vi "Get All VIs from Project.vi"(8 "error in (no error)":errorcluster, 11 "Project Path":path) -> (0 "error out":errorcluster, 2 "VI Virtual Paths":string[](array[string]), 3 "Project VIs":path[](array[path]), 5 "Project Name":string)   [LabVIEW 2015, in "SET Project Editor.lvlib"]
doc: "Get All VIs from Project.vi\n\nGet Paths (relative to project root) and Virtual Paths of project VIs\n\nExcluded VIs:\n- Password Protected VIs\n- vi.lib VIs\n- user.lib VIs\n- VIs of type other than Standard or Global"
uses:
  SET Project Editor.lvlib
panel:
  # "Get All VIs from Project.vi\n\nGet Paths (relative to project root) and Virtual Paths of project VIs\n\nExcluded VIs:\n- Password Protected VIs\n- vi.lib VIs\n- user.lib VIs\n- VIs of type other than Standard or Global"
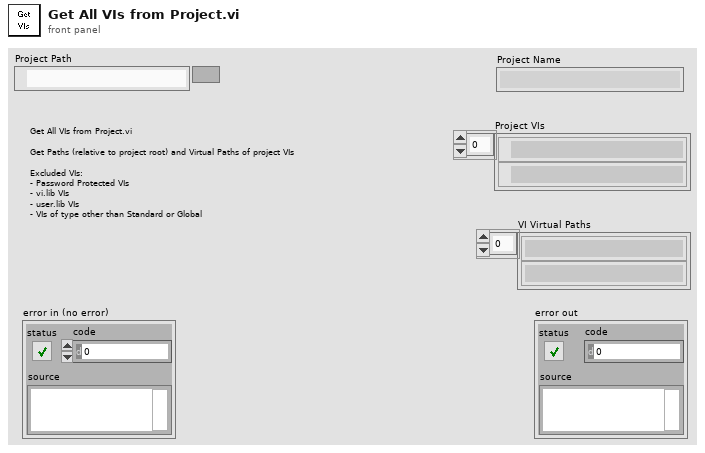
[diagram p1: front panel]
types:
  T1 = enum32{"invalid lock state", "Not Locked", "Locked (No Password)", "Password-protected"}
  T2 = enum32{"invalid VI type", "Standard VI", "Control VI", "Global VI", "Polymorphic VI", "Configuration VI", "SubSystem", "Facade VI", "Method VI", "Statechart Diagram VI"}
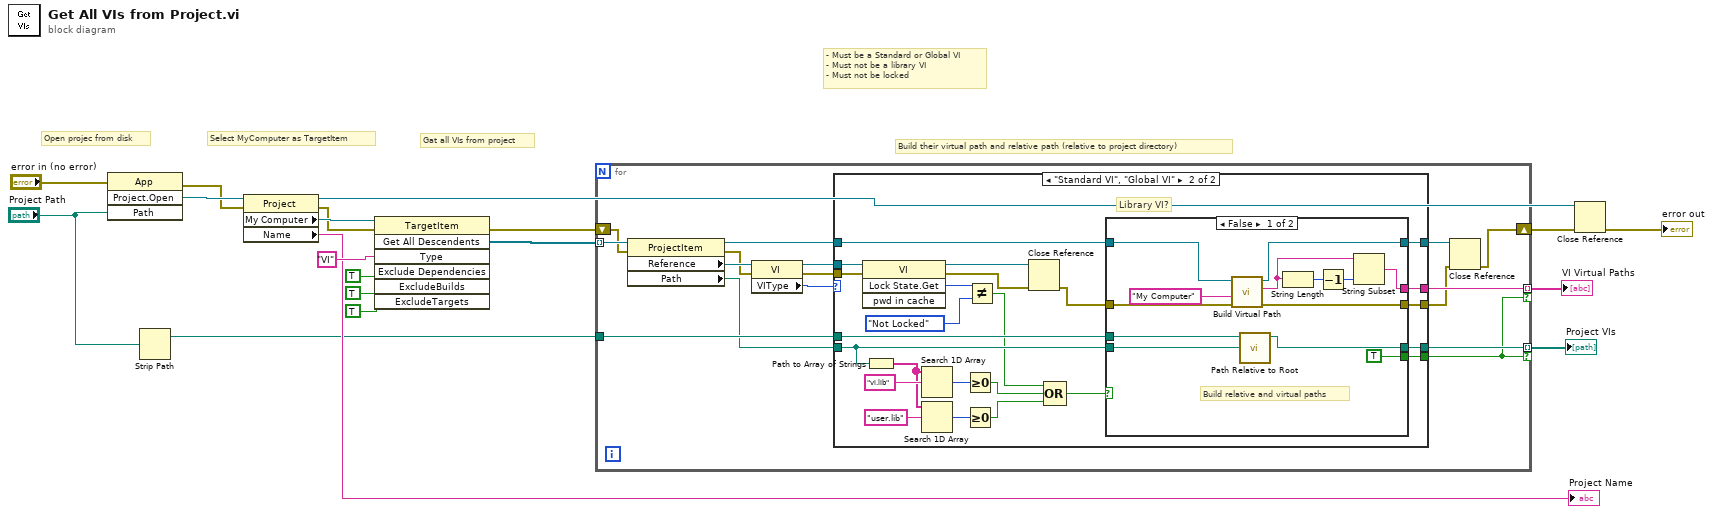
[diagram p0: block diagram]
diagram:
  # "- Must be a Standard or Global VI\n- Must not be a library VI\n- Must not be locked"
  # "Build their virtual path and relative path (relative to project directory)"
  # "Gat all VIs from project"
  # "Select MyComputer as TargetItem"
  # "Open projec from disk"
  n1 = invoke class="App" method="Project.Open"(error in="error in (no error)", "Path"="Project Path") -> (error out=w12:errorcluster, "Project:Open"=w15:refnum<vi>)  [unwired: 2 in, 2 out]
  n2 = Strip Path(path="Project Path") -> (stripped path=w3:path)  [unwired: 1 out]
  n3 = property class="Project"(reference=w15, error in=w12) -> (reference out=w6:refnum<vi>, error out=w11:errorcluster, "My Computer"=w14:refnum<vi>, "Name"=→"Project Name":string)
  n4 = invoke class="TargetItem" method="Get All Descendents"(reference=w14, error in=w11, "Type"="VI", "Exclude Dependencies"=TRUE ("ExcludeDependencies"), "ExcludeBuilds"=TRUE, "ExcludeTargets"=TRUE) -> (error out=w9:errorcluster, "All Descendents"=w10:refnum<vi>[])  [unwired: 1 in, 5 out]
  n5 = for {
    tunnel: w10 -> [w32] mode=indexing
    shift-right: [w22] -> w7
    shift-left: w9 -> [w29]
    tunnel: w3 -> [w35]
    tunnel: [w34] -> w2 mode=indexing if=w27
    tunnel: [w33] -> w1 mode=indexing if=w27
    n6 = property class="ProjectItem"(reference=w32, error in=w29) -> (reference out=w30:refnum<vi>, error out=w28:errorcluster, "Reference"=w31:refnum<vi>, "Path"=w25:path)
    n7 = property class="VI"(reference=w31, error in=w28) -> (reference out=w21:refnum<vi>, error out=w20:errorcluster, "VIType"=w26:T2)
    n8 = case shown="\"Standard VI\", \"Global VI\"" w26 {
      tunnel: [w36 w56] -> w23
      tunnel: w35 -> [_ w61]
      tunnel: [_ w60] -> w34
      tunnel: [_ w59] -> w33
      tunnel: w30 -> [w37 w57]
      tunnel: w20 -> [w36 w53]
      tunnel: [_ w58] -> w27
      tunnel: w25 -> [_ w40]
      tunnel: [w37 w55] -> w24
      tunnel: w21 -> [_ w54]
      frame "invalid VI type", Default {
      }
      frame "Standard VI", "Global VI" {
        # "Library VI?"
        n9 = invoke class="VI" method="Lock State.Get"(reference=w54, error in=w53) -> (reference out=w43:refnum<vi>, error out=w42:errorcluster, "Get Lock State"=w52:T1)  [unwired: 2 in, 1 out]
        n10 = Path to Array of Strings(0:w40) -> (2:w48:string[])  [unwired: 1 out]
        n11 = Search 1D Array(1D array=w48, element="vi.lib") -> (index of element=w47:i32)  [unwired: 1 in]
        n12 = Search 1D Array(1D array=w48, element="user.lib") -> (index of element=w46:i32)  [unwired: 1 in]
        n13 = Greater Or Equal To 0?(x=w47) -> (x >= 0?=w45:bool)
        n14 = Greater Or Equal To 0?(x=w46) -> (x >= 0?=w44:bool)
        n15 = Not Equal?(x=w52, y=T1."Not Locked" ("Lock State:Get")) -> (x != y?=w39:bool)
        n16 = Close Reference(reference=w43, error in (no error)=w42) -> (error out=w41:errorcluster)
        n17 = Compound Arithmetic op=OR(w39, w45, w44) -> (w38:bool)
        n18 = case shown="False" w38 {
          tunnel: w61 -> [w64 _]
          tunnel: [w62 _] -> w60
          tunnel: [w70 _] -> w59
          tunnel: [TRUE _] -> w58
          tunnel: w57 -> [w68 w76]
          tunnel: w40 -> [w63 _]
          tunnel: w41 -> [w67 w75]
          tunnel: [w65 w76] -> w55
          tunnel: [w66 w75] -> w56
          frame False {
            # "Build relative and virtual paths"
            n19 = call "Build Virtual Path.vi"("ProjItem* in"=w68, "Top Level Name"="My Computer", "error in (no error)"=w67) -> ("ProjItem* out"=w65:refnum<vi>, "VI ProjPath out"=w71:string, "error out"=w66:errorcluster)  [unwired: 5 in]
            n20 = call "Path Relative to Root.vi"("ItemPath"=w63, "RootDir"=w64) -> ("ItemPath (Relative to Root)"=w62:path)  [unwired: 9 in]
            n21 = String Length(string=w71) -> (length=w73:i32)
            n22 = Decrement(x=w73) -> (x-1=w72:i32)
            n23 = String Subset(string=w71, length (rest)=w72) -> (substring=w70:string)  [unwired: 1 in]
          }
          frame True {
          }
        }
      }
    }
    n24 = Close Reference(reference=w24, error in (no error)=w23) -> (error out=w22:errorcluster)
  }
  "Project VIs" <- w2
  "VI Virtual Paths" <- w1
  n25 = Close Reference(reference=w6, error in (no error)=w7) -> (error out=→"error out":errorcluster)
